vi "Write Serial Session.vi"(8 "error in (no error)":errorcluster, 10 "Session Handle":T1, 11 "CR5 in":refnum<class "CR5.lvclass">) -> (0 "error out":errorcluster, 3 "CR5 out":refnum<class "CR5.lvclass">)   [LabVIEW 2015, in "CR5.lvclass"]
uses:
  CR5.lvclass
  <userlib>/_Session Fwk/Typedefs/Session Handle.ctl
  <userlib>/_Session Fwk/Session - Root.lvclass
  CR5.lvclass/CR5.ctl
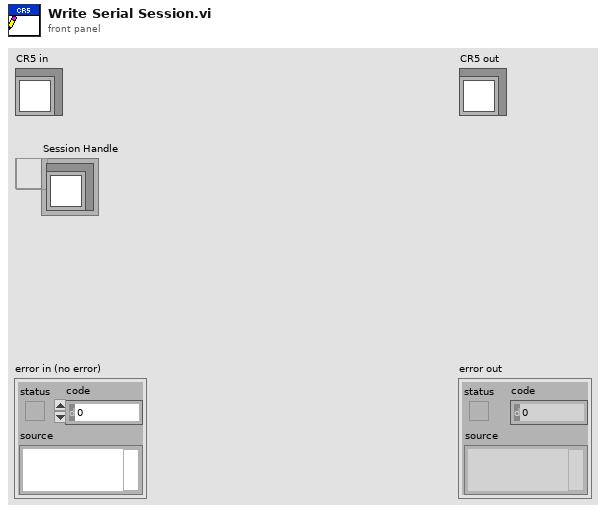
[diagram p1: front panel]
types:
  T1 = typedef "Session - Root.lvclass/Session Handle.ctl" = refnum<data-value>
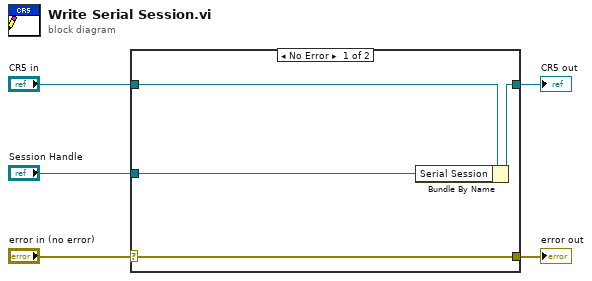
[diagram p0: block diagram]
diagram:
  n1 = case shown="No Error" "error in (no error)" {
    selector: "error in (no error)" -> [w9 w10]
    tunnel: [w9 w10] -> w4
    tunnel: [w7 w11] -> w2
    tunnel: "CR5 in" -> [w8 w11]
    tunnel: "Session Handle" -> [w6 _]
    frame No Error {
      n2 = Bundle By Name(cluster=w8, "Serial Session"=w6) -> (w7:refnum<class "CR5.lvclass">)
    }
    frame Error {
    }
  }
  "error out" <- w4
  "CR5 out" <- w2
